vi "S2C_Access_Fetch.vi"(8 "Error In":errorcluster, 11 "Query":string) -> (0 "Error Out":errorcluster, 3 "Data":string)   [LabVIEW 2015]
uses:
  S2C_Access_Globals.vi
  <vilib>/addons/database/Connection.llb/Conn Execute.vi
  <vilib>/addons/database/Recordset.llb/Rec Fetch Recordset Data (R).vi
  <vilib>/addons/database/Recordset.llb/Rec Destroy - Connection.vi
  <vilib>/addons/database/_DB Variant To Data/Database Variant To Data.xnode
  <vilib>/addons/database/NI_Database_API.lvlib
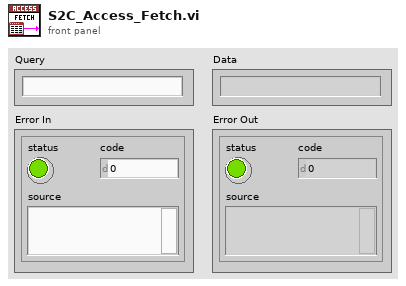
[diagram p1: front panel]
types:
  T1 = typedef "NI_Database_API.lvlib/Conn ObjectReference.ctl" = refnum<k1>
  T2 = typedef "NI_Database_API.lvlib/Rec ObjectReference.ctl" = refnum<k1>
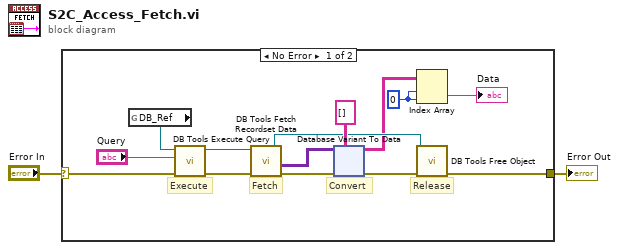
[diagram p0: block diagram]
diagram:
  n1 = case shown="No Error" "Error In" {
    selector: "Error In" -> [w9 w61]
    tunnel: [w8 w61] -> w1
    frame No Error {
      w4 = 0 ("disabled index (col)")
      # "Release"
      # "Fetch"
      # "Execute"
      # "Convert"
      n2 = global read "S2C_Access_Globals.vi" "DB_Ref"() -> (w7:T1)
      n3 = call-poly <vilib>:"DB Tools Execute Query.vi"("error in (no error)"=w9, "SQL query"="Query", "connection reference"=w7) -> ("error out"=w11:errorcluster, "recordset reference"=w10:T2)  [unwired: 5 in]
      n4 = call-poly <vilib>:"DB Tools Fetch Recordset Data.vi"("error in (no error)"=w11, "recordset reference"=w10) -> ("error out"=w16:errorcluster, "recordset data"=w15:variant[][], "recordset reference out"=w12:T2)  [unwired: 3 in]
      n5 = xnode "Database Variant To Data"("database variant"=w15, "error in (no error)"=w16, "type"=string[][] []) -> ("data"=w5:string[][], "error out"=w14:errorcluster)
      n6 = Index Array(array=w5, index (row)=w4, index (col)=w4) -> (element=→"Data":string)
      n7 = call-poly <vilib>:"DB Tools Free Object.vi"("error in (no error)"=w14, "recordset reference"=w12) -> ("error out"=w8:errorcluster)  [unwired: 8 in, 1 out]
    }
    frame Error {
    }
  }
  "Error Out" <- w1
